vi "Documentation.vi"() -> (0 "Author":string, 1 "History":string, 2 "Version":string, 3 "Description":string)   [LabVIEW 2021, in "Template_Plugin.lvlib"]
uses:
  Template_Plugin.lvlib
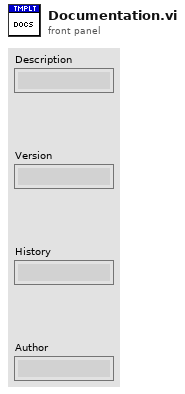
[diagram p1: front panel]
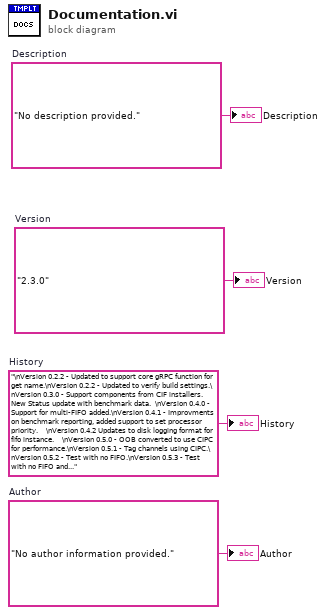
[diagram p0: block diagram]
diagram:
  w1 = "No author information provided."  # Author
  w2 = "\nVersion 0.2.2 - Updated to support core gRPC function for get name.\nVersion 0.2.2 - Updated to verify build settings.\nVersion 0.3.0 - Support components from CIF installers.  New Status update with benchmark data.  \nVersion 0.4.0 - Support for multi-FIFO added.\nVersion 0.4.1 - Improvments on benchmark reporting, added support to set processor priority.    \nVersion 0.4.2 Updates to disk logging format for fifo instance.    \nVersion 0.5.0 - OOB converted to use CIPC for performance.\nVersion 0.5.1 - Tag channels using CIPC.\nVersion 0.5.2 - Test with no FIFO.\nVersion 0.5.3 - Test with no FIFO and NI_Chan.\nVersion 0.5.4 - Test with no FIFO, modified CIPC for single call.\nVersion 0.6.0 - Support for CIPC FIFO channels.\nVersion 2.0.0 - Version alignment with UIVersion 2.1.0.0 Built using automated script.Version 2.2.0.0 Built using automated script.\n\nVersion 2.2.0.8 notes\n\nVersion 2.2.0.9 notes\nVersion 2.2.0.10 notes\nVersion 2.2.0.11 notes\nVersion 2.2.0.12 notes\nVersion 2.2.0.17 test of automated build\rVersion 2.3.0.18 - This is a test\nVersion 0.2.2 - Updated to support core gRPC function for get name.\nVersion 0.2.2 - Updated to verify build settings.\nVersion 0.3.0 - Support components from CIF installers.  New Status update with benchmark data.  \nVersion 0.4.0 - Support for multi-FIFO added.\nVersion 0.4.1 - Improvments on benchmark reporting, added support to set processor priority.    \nVersion 0.4.2 Updates to disk logging format for fifo instance.    \nVersion 0.5.0 - OOB converted to use CIPC for performance.\nVersion 0.5.1 - Tag channels using CIPC.\nVersion 0.5.2 - Test with no FIFO.\nVersion 0.5.3 - Test with no FIFO and NI_Chan.\nVersion 0.5.4 - Test with no FIFO, modified CIPC for single call.\nVersion 0.6.0 - Support for CIPC FIFO channels.\nVersion 2.0.0 - Version alignment with UIVersion 2.1.0.0 Built using automated script.Version 2.2.0.0 Built using automated script.\n\nVersion 2.2.0.8 notes\n\nVersion 2.2.0.9 notes\nVersion 2.2.0.10 notes\nVersion 2.2.0.11 notes\nVersion 2.2.0.12 notes\nVersion 2.2.0.17 test of automated build\nVersion 2.3.0.18 - This is a test\rVersion 2.3.0.19 - This is a test"  # History
  w3 = "2.3.0"  # Version
  w4 = "No description provided."  # Description
  "Description" <- w4
  "Version" <- w3
  "History" <- w2
  "Author" <- w1
